vi "Get Port.vi"(8 "error in (no error)":errorcluster, 11 "LakeShore.340 in":refnum<class "LakeShore.340.lvclass">) -> (0 "error out":errorcluster, 2 "port":u32, 3 "LakeShore.340 out":refnum<class "LakeShore.340.lvclass">)   [LabVIEW 2016, in "LakeShore.340.lvclass"]
uses:
  LakeShore.340.lvclass
  <userlib>/LevyLab/Levylab Instruments/SMOs/Instrument/Instrument.lvclass
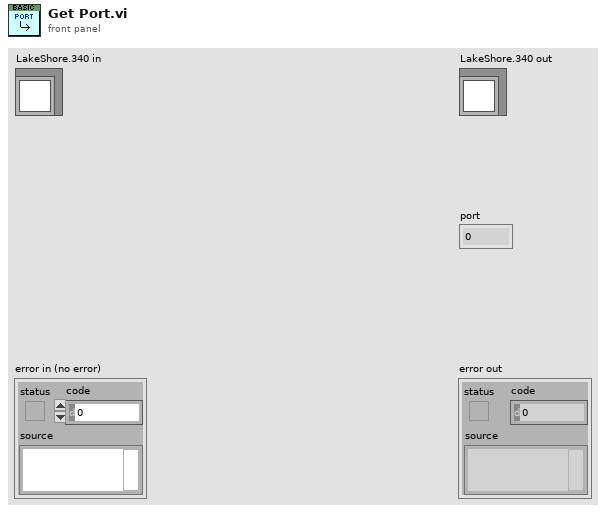
[diagram p1: front panel]
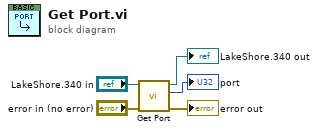
[diagram p0: block diagram]
diagram:
  n1 = call-parent "Get Port.vi"("error in (no error)"="error in (no error)", "Instrument in"="LakeShore.340 in") -> ("error out"=→"error out":errorcluster, "port"=→"port":u32, "Instrument out"=→"LakeShore.340 out":refnum<class "LakeShore.340.lvclass">)  [unwired: 7 in]
